vi "zoom_or_move_to_roi_grMD.vi"() -> ()   [LabVIEW 2017]
doc: "SciScan 1.2 160622"
uses:
  Custom Controls/pixel resolution enum.ctl
  GFG/GFGDisplayRefsGet.vi
  GFG/GFGfpRefGet.vi
  GFG/GFG library.lvlib
  GFG/GFGbooleanGet.vi
panel:
  out "error out 2":errorcluster
  out "error out":errorcluster
  in  "error in (no error)":errorcluster
  in  "stop":bool
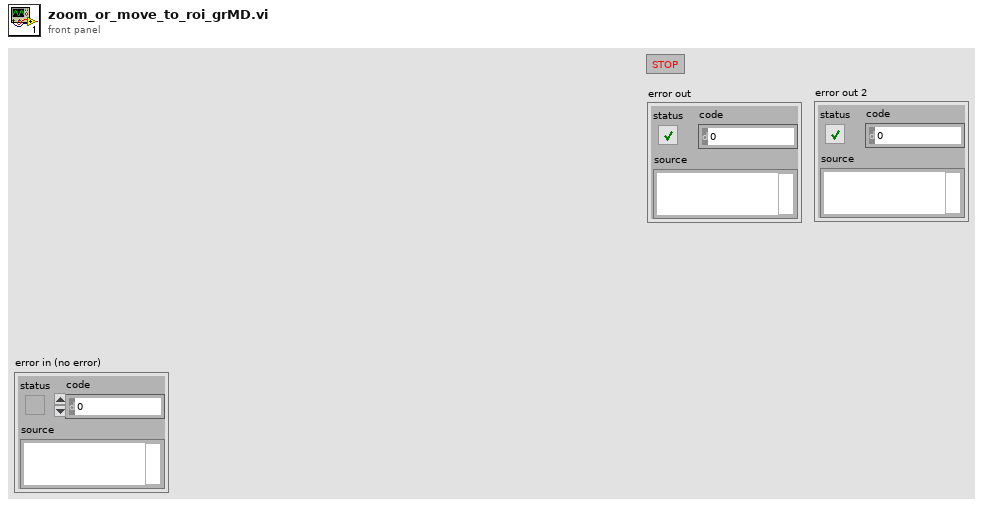
[diagram p1: front panel]
types:
  T1 = cluster{"Global Rectangle":i32[], "Contours":cluster{"Contour Type":u32, "ROI Type":u32, "Points":i32[]}[]}
  T2 = enum16{"Left Button", "Center Button", "Right Button", "Window Close"}
  T3 = cluster{"Channel 1 small":refnum<vi>, "Channel 2 small":refnum<vi>, "Channel 3 small":refnum<vi>, "Channel 4 small":refnum<vi>, "Channel 1 large":refnum<vi>, "Channel 2 large":refnum<vi>, "Channel 3 large":refnum<vi>, "Channel 4 large":refnum<vi>, "RGB overlay":refnum<vi>, "ROI Image display":refnum<vi>, "arb line scan display":refnum<vi>, "Channel 5 large":refnum<vi>}
  T4 = enum8{"Enabled", "Disabled", "Disabled and Grayed Out"}
  T5 = typedef "pixel resolution enum.ctl" = enum16{"128 x 128", "256 x 128", "256 x 256", "512 x  64", "512 x 128", "512 x 256", "512 x 512", "1024 x 512", "1024 x 1024", "arbitrary"}
  T6 = cluster{"WaveformChartRef":refnum<vi>, "DigitalRef":refnum<vi>, "ArrayRef":refnum<vi>, "TabControlRef":refnum<vi>, "EnumRef":refnum<vi>, "RingRef":refnum<vi>, "BooleanRef":refnum<vi>, "KnobRef":refnum<vi>, "SlideRef":refnum<vi>, "PathRef":refnum<vi>, "StringRef":refnum<vi>, "ComboBox":refnum<vi>, "WaveformGraphRef":refnum<vi>}
  T7 = typedef "ROI Descriptor" = cluster{"Global Rectangle":i32[], "Contours":cluster{"ID":enum32{"External", "Internal"}, "Type":u32, "Coordinates":i32[]}[]}
  T8 = cluster{"ID":enum32{"External", "Internal"}, "Type":u32, "Coordinates":i32[]}[]
  T9 = cluster{"ID":enum32{"External", "Internal"}, "Type":u32, "Coordinates":i32[]}
  T10 = cluster{"pixel resolution":variant, "x offset":variant, "x pixel size":variant, "y offset":variant, "y pixel size":variant, "y pixels":variant}
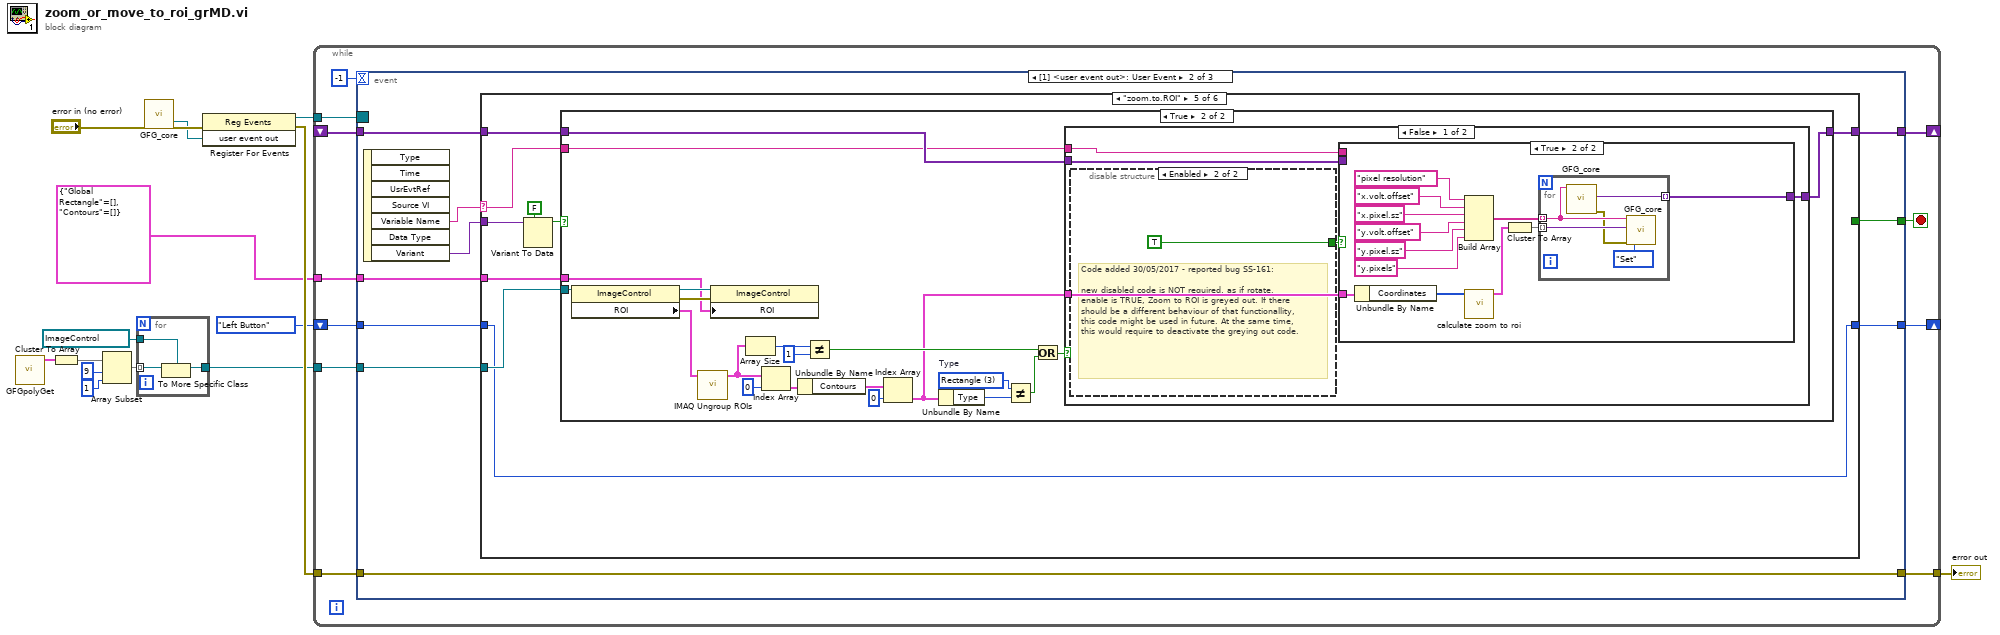
[diagram p0: block diagram]
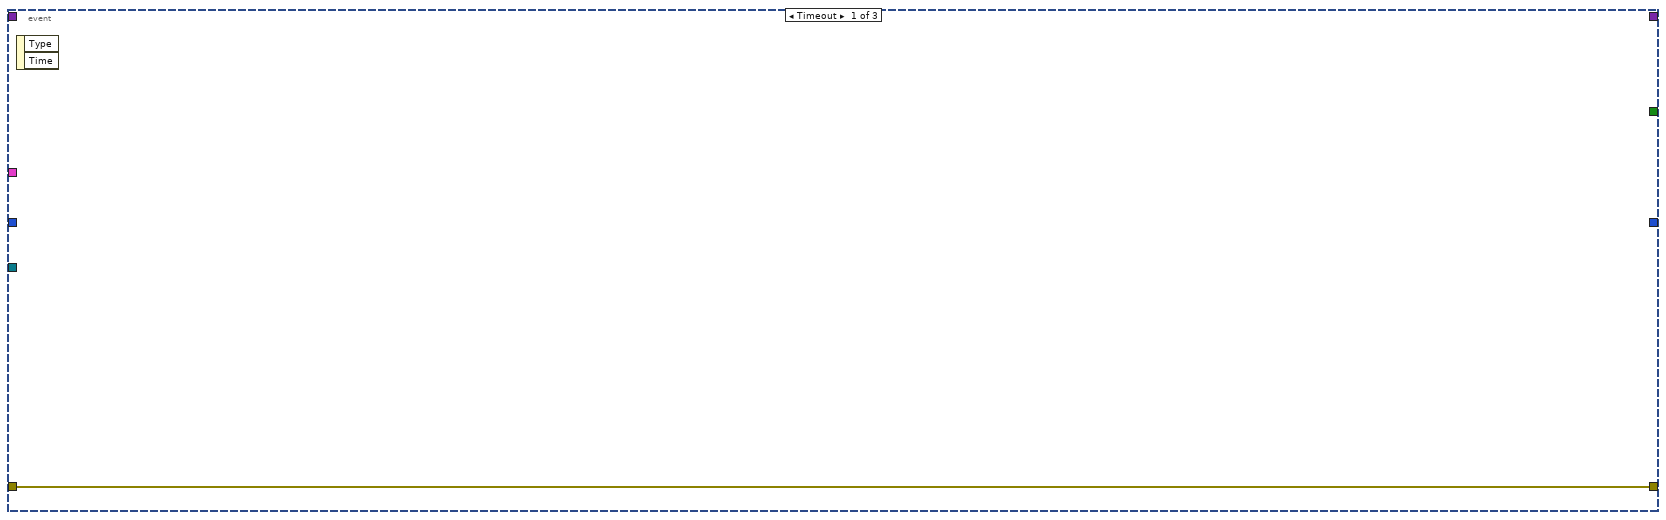
[diagram p2: hidden frame]
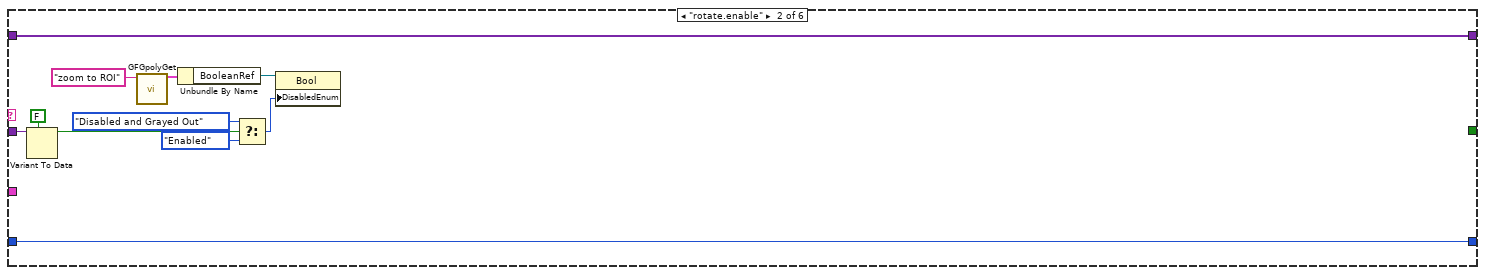
[diagram p4: hidden frame]
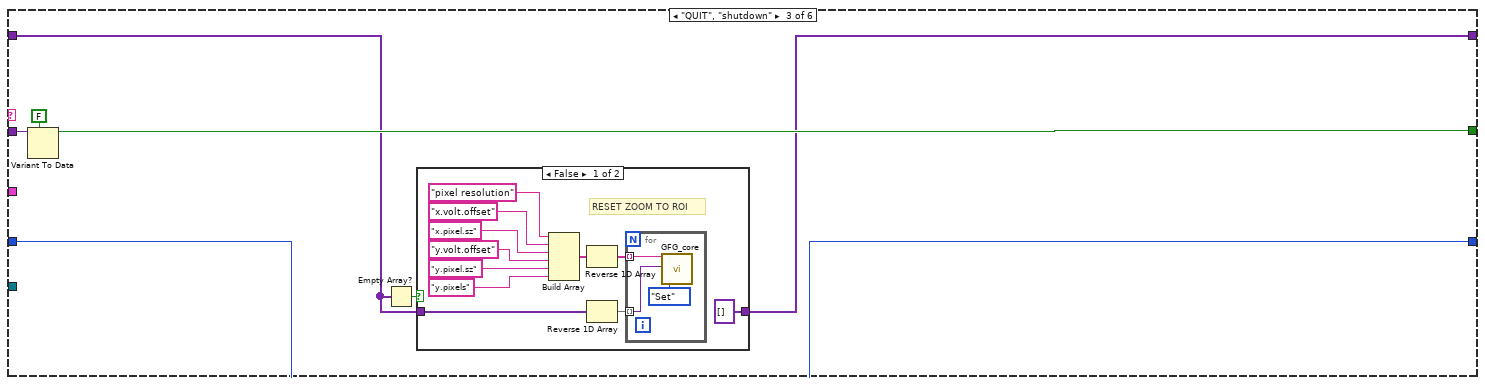
[diagram p5: hidden frame]
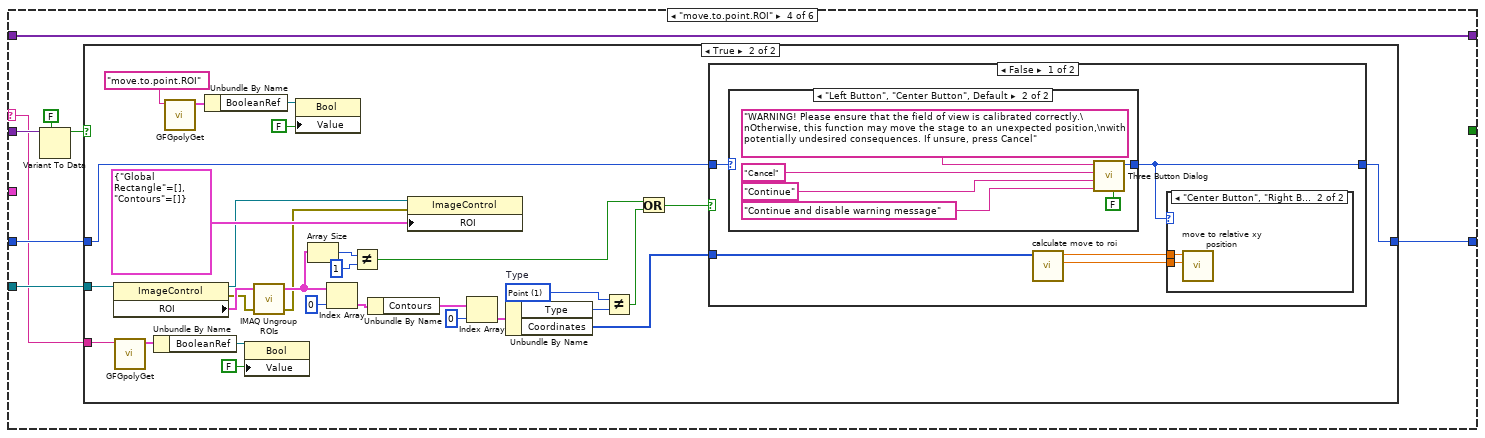
[diagram p7: hidden frame]
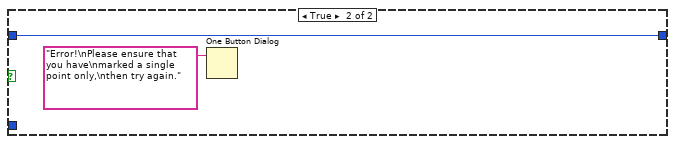
[diagram p11: hidden frame]
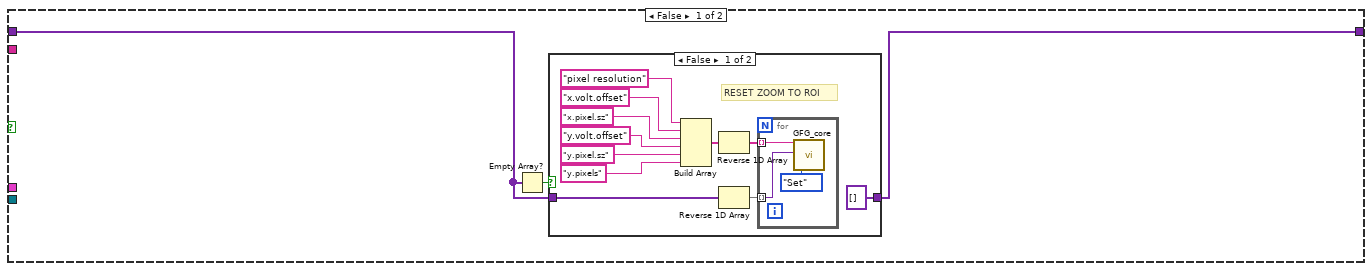
[diagram p12: hidden frame]
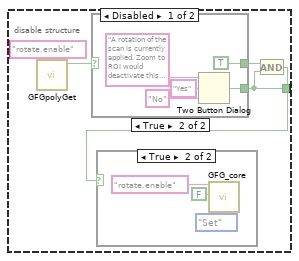
[diagram p14: hidden frame]
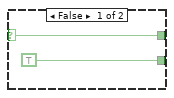
[diagram p16: hidden frame]
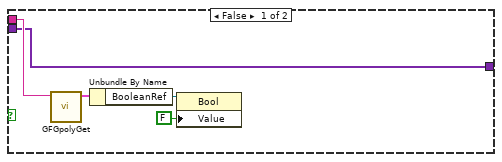
[diagram p17: hidden frame]
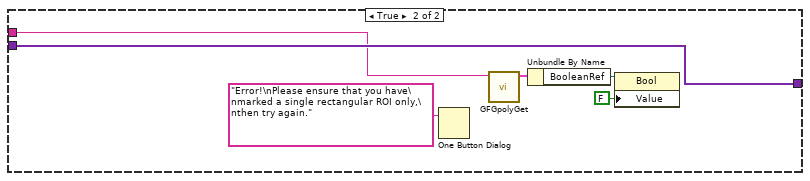
[diagram p18: hidden frame]
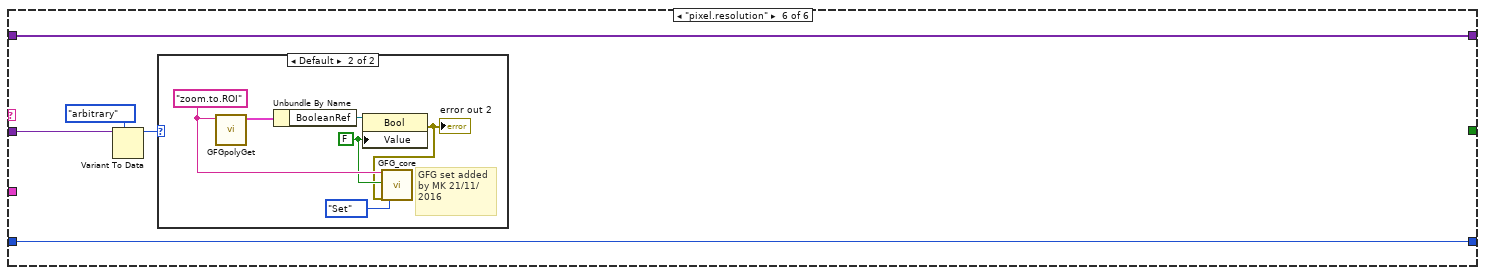
[diagram p19: hidden frame]
diagram:
  n1 = call-poly "GFGpolyGet.vi"() -> ("DisplayRefsOut(generic class)"=w10:T3)  [unwired: 10 in, 1 out]
  n2 = Cluster To Array(cluster=w10) -> (array=w13:refnum<vi>[])
  n3 = Array Subset(array=w13, index=9, length=1) -> (w12:refnum<vi>[])
  n4 = for {
    tunnel: w12 -> [w18] mode=indexing
    tunnel: refnum<vi> refnum ("arbitrary line scan display") -> [w17]
    tunnel: [w16] -> w3
    n5 = To More Specific Class(target class=w17, reference=w18) -> (specific class reference=w16:refnum<vi>)  [unwired: 1 in, 1 out]
  }
  n6 = call "GFG_core.vi"("error in (no error)"="error in (no error)") -> ("user event out"=w5:refnum<user-event>, "error out"=w6:errorcluster)  [unwired: 12 in, 5 out]
  n7 = register-events(error in=w6, w5) -> (reference out=w4:refnum<event-registration>, error out=w8:errorcluster)  [unwired: 1 in]
  n8 = while {
    tunnel: w4 -> [w29]
    tunnel: w8 -> [w27]
    tunnel: [w26] -> w9
    tunnel: w3 -> [w24]
    shift-right: [w23] -> _
    shift-left: _ -> [w22]
    shift-right: [w20] -> _
    shift-left: T2."Left Button" ("Which Button?") -> [w21]
    tunnel: T1 {"Global Rectangle"=[], "Contours"=[]} ("ROI") -> [w19]
    stop <- w28 stop-if-true
    n9 = event shown="[1] <user event out>: User Event" {
      selector: w29 -> [_ _ _]
      dyn-events: _ -> [_ _ _]
      timeout: -1 -> [_ _ _]
      tunnel: [_ w38 _] -> w28
      tunnel: w27 -> [w30 w37 _]
      tunnel: [w30 w37 _] -> w26
      tunnel: w24 -> [_ w36 _]
      tunnel: [_ w35 _] -> w23
      tunnel: w22 -> [_ w34 _]
      tunnel: w21 -> [_ w33 _]
      tunnel: [_ w32 _] -> w20
      tunnel: w19 -> [_ w31 _]
      event Timeout {
        n10 = event-data() -> ()  [unwired: 1 in, 2 out]
      }
      event User Event {
        n11 = event-data() -> ("Variable Name"=w40:string, "Variant"=w39:variant)  [unwired: 1 in, 5 out]
        n12 = case shown="\"zoom.to.ROI\"" w40 {
          selector: w40 -> [_ _ _ w76 w133 _]
          tunnel: w39 -> [_ w46 w60 w80 w136 w232]
          tunnel: [_ _ w58 _ _ _] -> w38
          tunnel: w36 -> [_ _ _ w83 w139 _]
          tunnel: [w42 w43 w57 w82 w138 w229] -> w35
          tunnel: w34 -> [w42 w43 w55 w82 w137 w229]
          tunnel: w33 -> [w41 w53 w56 w78 w132 w228]
          tunnel: [w41 w53 w56 w77 w132 w228] -> w32
          tunnel: w31 -> [_ _ _ _ w131 _]
          frame "False", Default {
          }
          frame "rotate.enable" {
            n13 = Variant To Data(type=FALSE, Variant=w46) -> (data=w44:bool)  [unwired: 1 in, 1 out]
            n14 = call-poly "GFGpolyGet.vi"("Variable Name in"="zoom to ROI") -> ("output cluster"=w51:T6)  [unwired: 9 in, 1 out]
            n15 = Unbundle By Name(w51) -> ("BooleanRef"=w50:refnum<vi>)
            n16 = Select(t=T4."Disabled and Grayed Out" ("Disabled"), s=w44, f=T4."Enabled" ("Disabled")) -> (s? t:f=w49:T4)
            n17 = property class="Bool"(reference=w50, "DisabledEnum"=w49) -> ()  [unwired: 1 in, 2 out]
          }
          frame "QUIT", "shutdown" {
            n18 = Variant To Data(type=FALSE ("want seconds? (F)"), Variant=w60) -> (data=w58:bool)  [unwired: 1 in, 1 out]
            n19 = Empty Array?(array=w55) -> (empty?=w54:bool)
            n20 = case shown="False" w54 {
              tunnel: [variant[] [] w75] -> w57
              tunnel: w55 -> [w62 w75]
              frame False {
                # "RESET ZOOM TO ROI"
                n21 = Build Array("pixel resolution" ("Variable Name in"), "x.volt.offset" ("Variable Name in"), "x.pixel.sz" ("Variable Name in"), "y.volt.offset" ("Variable Name in"), "y.pixel.sz" ("Variable Name in"), "y.pixels" ("Variable Name in")) -> (w63:string[])
                n22 = Reverse 1D Array(array=w63) -> (reversed array=w71:string[])
                n23 = Reverse 1D Array(array=w62) -> (reversed array=w70:variant[])
                n24 = for {
                  tunnel: w71 -> [w73] mode=indexing
                  tunnel: w70 -> [w72] mode=indexing
                  n25 = call "GFG_core.vi"("Variable Name in"=w73, "Variant in"=w72, "Action"=enum16{"Init", "Set", "Get", "Clear"}."Set") -> ()  [unwired: 10 in, 7 out]
                }
              }
              frame True {
                # "Do nothing, as the zoom to ROI hasn't been used yet."
              }
            }
          }
          frame "move.to.point.ROI" {
            n26 = Variant To Data(type=FALSE, Variant=w80) -> (data=w79:bool)  [unwired: 1 in, 1 out]
            n27 = case shown="True" w79 {
              tunnel: w83 -> [_ w114]
              tunnel: w78 -> [w84 w98]
              tunnel: [w84 w97] -> w77
              tunnel: w76 -> [_ w85]
              frame False {
              }
              frame True {
                w101 = u32 1 items=["No Selection", "Point", "Line", "Rectangle", "Oval", "Polygon", "Freehand Region", "Annulus", "Unused2", "Unused3", "Broken Line", "Freehand Line", "Rotated Rectangle"]  # Type
                n28 = property class="ImageControl"(reference=w114) -> (reference out=w91:refnum<vi>, error out=w90:errorcluster, "ROI"=w113:T1)  [unwired: 1 in]
                n29 = call-poly "GFGpolyGet.vi"("Variable Name in"=w85) -> ("output cluster"=w88:T6)  [unwired: 9 in, 1 out]
                n30 = Unbundle By Name(w88) -> ("BooleanRef"=w87:refnum<vi>)
                n31 = call-poly "GFGpolyGet.vi"("Variable Name in"="move.to.point.ROI") -> ("output cluster"=w95:T6)  [unwired: 9 in, 1 out]
                n32 = Unbundle By Name(w95) -> ("BooleanRef"=w94:refnum<vi>)
                n33 = property class="Bool"(reference=w87, "Value"=FALSE ("true")) -> ()  [unwired: 1 in, 2 out]
                n34 = call "IMAQ Ungroup ROIs"("error in (no error)"=w90, "ROI Descriptor"=w113) -> ("error out"=w89:errorcluster, "ROI Descriptors out"=w108:T7[])  [unwired: 2 in]
                n35 = property class="Bool"(reference=w94, "Value"=FALSE) -> ()  [unwired: 1 in, 2 out]
                n36 = Array Size(array=w108) -> (size(s)=w112:i32)
                n37 = Index Array(array=w108, index=0) -> (element=w106:T7)
                n38 = Not Equal?(x=w112, y=1) -> (x != y?=w110:bool)
                n39 = Unbundle By Name(w106) -> ("Contours"=w104:T8)
                n40 = property class="ImageControl"(reference=w91, error in=w89, "ROI"=T1 {"Global Rectangle"=[], "Contours"=[]}) -> ()  [unwired: 2 out]
                n41 = Index Array(array=w104, index=0) -> (element=w103:T9)
                n42 = Unbundle By Name(w103) -> ("Type"=w102:u32, "Coordinates"=w99:i32[])
                n43 = Not Equal?(x=w101, y=w102) -> (x != y?=w100:bool)
                n44 = Or(x=w110, y=w100) -> (x .or. y?=w109:bool)
                n45 = case shown="False" w109 {
                  tunnel: w99 -> [w119 _]
                  tunnel: w98 -> [w118 w129]
                  tunnel: [w115 w129] -> w97
                  frame False {
                    n46 = case shown="\"Left Button\", \"Center Button\", Default" w118 {
                      selector: w118 -> [w120 _]
                      tunnel: [w120 w123] -> w115
                      frame "Right Button" {
                      }
                      frame "Left Button", "Center Button", Default {
                        n47 = call <vilib>:"Three Button Dialog.vi"("Allow user to close window? (TRUE)"=FALSE, "Right Button Text (\"Cancel\")"="Continue and disable warning message" ("Center Button Text (\"No\")"), "Center Button Text (\"No\")"="Continue" ("Left Button Text (\"Yes\")"), "Left Button Text (\"Yes\")"="Cancel" ("Right Button Text (\"Cancel\")"), "message"="WARNING! Please ensure that the field of view is calibrated correctly.\nOtherwise, this function may move the stage to an unexpected position,\nwith potentially undesired consequences. If unsure, press Cancel") -> ("Which Button?"=w123:T2)  [unwired: 6 in]
                      }
                    }
                    n48 = call "calculate move to roi.vi"("Coordinates"=w119) -> ("setY"=w116:dbl, "setX"=w117:dbl)  [unwired: 9 in]
                    n49 = case shown="\"Center Button\", \"Right Button\"" w115 {
                      tunnel: w117 -> [_ w128]
                      tunnel: w116 -> [_ w127]
                      frame "Left Button", Default {
                      }
                      frame "Center Button", "Right Button" {
                        n50 = call "move to relative xy position.vi"("setY"=w127, "setX"=w128) -> ()  [unwired: 10 in]
                      }
                    }
                  }
                  frame True {
                    n51 = One Button Dialog(message="Error!\nPlease ensure that you have\nmarked a single point only,\nthen try again.") -> ()  [unwired: 1 in, 1 out]
                  }
                }
              }
            }
          }
          frame "zoom.to.ROI" {
            n52 = Variant To Data(type=FALSE, Variant=w136) -> (data=w134:bool)  [unwired: 1 in, 1 out]
            n53 = case shown="True" w134 {
              tunnel: w139 -> [_ w178]
              tunnel: [w140 w163] -> w138
              tunnel: w137 -> [w141 w162]
              tunnel: w133 -> [_ w159]
              tunnel: w131 -> [_ w158]
              frame False {
                n54 = Empty Array?(array=w141) -> (empty?=w142:bool)
                n55 = case shown="False" w142 {
                  tunnel: [variant[] [] w157] -> w140
                  tunnel: w141 -> [w144 w157]
                  frame False {
                    # "RESET ZOOM TO ROI"
                    n56 = Build Array("pixel resolution" ("Variable Name in"), "x.volt.offset" ("Variable Name in"), "x.pixel.sz" ("Variable Name in"), "y.volt.offset" ("Variable Name in"), "y.pixel.sz" ("Variable Name in"), "y.pixels" ("Variable Name in")) -> (w145:string[])
                    n57 = Reverse 1D Array(array=w145) -> (reversed array=w153:string[])
                    n58 = Reverse 1D Array(array=w144) -> (reversed array=w152:variant[])
                    n59 = for {
                      tunnel: w153 -> [w155] mode=indexing
                      tunnel: w152 -> [w154] mode=indexing
                      n60 = call "GFG_core.vi"("Variable Name in"=w155, "Variant in"=w154, "Action"=enum16{"Init", "Set", "Get", "Clear"}."Set") -> ()  [unwired: 10 in, 7 out]
                    }
                  }
                  frame True {
                    # "Do nothing, as the zoom to ROI hasn't been used yet."
                  }
                }
              }
              frame True {
                w166 = u32 3 items=["No Selection", "Point", "Line", "Rectangle", "Oval", "Polygon", "Freehand Region", "Annulus", "Unused2", "Unused3", "Broken Line", "Freehand Line", "Rotated Rectangle"]  # Type
                n61 = property class="ImageControl"(reference=w178) -> (reference out=w161:refnum<vi>, error out=w160:errorcluster, "ROI"=w177:T1)  [unwired: 1 in]
                n62 = call "IMAQ Ungroup ROIs"("ROI Descriptor"=w177) -> ("ROI Descriptors out"=w172:T7[])  [unwired: 3 in, 1 out]
                n63 = property class="ImageControl"(reference=w161, error in=w160, "ROI"=w158) -> ()  [unwired: 2 out]
                n64 = Array Size(array=w172) -> (size(s)=w176:i32)
                n65 = Index Array(array=w172, index=0) -> (element=w170:T7)
                n66 = Unbundle By Name(w170) -> ("Contours"=w168:T8)
                n67 = Not Equal?(x=w176, y=1) -> (x != y?=w174:bool)
                n68 = Index Array(array=w168, index=0) -> (element=w164:T9)
                n69 = Unbundle By Name(w164) -> ("Type"=w167:u32)
                n70 = Not Equal?(x=w166, y=w167) -> (x != y?=w165:bool)
                n71 = Or(x=w174, y=w165) -> (x .or. y?=w173:bool)
                n72 = case shown="False" w173 {
                  tunnel: w164 -> [w183 _]
                  tunnel: [w182 w227] -> w163
                  tunnel: w162 -> [w179 w227]
                  tunnel: w159 -> [w180 w226]
                  frame False {
                    n73 = disable-structure shown="Enabled" {
                      disable-tunnel: [w185 TRUE ("T button?")] -> w181
                      frame Disabled {
                        n74 = call-poly "GFGpolyGet.vi"("Variable Name in"="rotate.enable" ("message")) -> ("Boolean Value OUT"=w187:bool)  [unwired: 9 in, 1 out]
                        n75 = case shown="True" w187 {
                          selector: w187 -> [w192 _]
                          tunnel: [TRUE ("T button?") w195] -> w185
                          tunnel: [w192 TRUE] -> w186
                          frame False {
                          }
                          frame True {
                            n76 = Two Button Dialog(message="A rotation of the scan is currently applied. Zoom to ROI would deactivate this rotation. Do you want to proceed?", 1:"No" ("F button name (\"Cancel\")"), 2:"Yes" ("T button name (\"OK\")")) -> (T button?=w195:bool)
                          }
                        }
                        n77 = And(x=w186, y=w185) -> (x .and. y?=w184:bool)
                        n78 = case shown="True" w184 {
                          frame False {
                          }
                          frame True {
                            n79 = call "GFG_core.vi"("Variable Name in"="rotate.enable" ("message"), "Variant in"=FALSE ("T button?"), "Action"=enum16{"Init", "Set", "Get", "Clear"}."Set") -> ()  [unwired: 10 in, 7 out]
                          }
                        }
                      }
                      frame Enabled {
                        # "Code added 30/05/2017 - reported bug SS-161:\n\nnew disabled code is NOT required, as if rotate.enable is TRUE, Zoom to ROI is greyed out. If there should be a different behaviour of that functionallity, this code might be used in future. At the same time, this would require to deactivate the greying out code."
                      }
                    }
                    n80 = case shown="True" w181 {
                      tunnel: w183 -> [_ w216]
                      tunnel: [w200 w215] -> w182
                      tunnel: w180 -> [w201 _]
                      tunnel: w179 -> [w200 _]
                      frame False {
                        n81 = call-poly "GFGpolyGet.vi"("Variable Name in"=w201) -> ("output cluster"=w204:T6)  [unwired: 9 in, 1 out]
                        n82 = Unbundle By Name(w204) -> ("BooleanRef"=w203:refnum<vi>)
                        n83 = property class="Bool"(reference=w203, "Value"=FALSE ("true")) -> ()  [unwired: 1 in, 2 out]
                      }
                      frame True {
                        n84 = Unbundle By Name(w216) -> ("Coordinates"=w214:i32[])
                        n85 = Build Array("pixel resolution" ("Variable Name in"), "x.volt.offset" ("Variable Name in"), "x.pixel.sz" ("Variable Name in"), "y.volt.offset" ("Variable Name in"), "y.pixel.sz" ("Variable Name in"), "y.pixels" ("Variable Name in")) -> (w207:string[])
                        n86 = call "calculate zoom to roi.vi"("Coordinates"=w214) -> ("output cluster"=w208:T10)  [unwired: 10 in]
                        n87 = Cluster To Array(cluster=w208) -> (array=w206:variant[])
                        n88 = for {
                          tunnel: w207 -> [w219] mode=indexing
                          tunnel: w206 -> [w220] mode=indexing
                          tunnel: [w218] -> w215 mode=indexing
                          n89 = call "GFG_core.vi"("Variable Name in"=w219) -> ("Variant Out"=w218:variant, "error out"=w217:errorcluster)  [unwired: 12 in, 5 out]
                          n90 = call "GFG_core.vi"("Variable Name in"=w219, "Variant in"=w220, "error in (no error)"=w217, "Action"=enum16{"Init", "Set", "Get", "Clear"}."Set") -> ()  [unwired: 9 in, 7 out]
                        }
                      }
                    }
                  }
                  frame True {
                    n91 = One Button Dialog(message="Error!\nPlease ensure that you have\nmarked a single rectangular ROI only,\nthen try again.") -> ()  [unwired: 1 in, 1 out]
                    n92 = call-poly "GFGpolyGet.vi"("Variable Name in"=w226) -> ("output cluster"=w225:T6)  [unwired: 9 in, 1 out]
                    n93 = Unbundle By Name(w225) -> ("BooleanRef"=w224:refnum<vi>)
                    n94 = property class="Bool"(reference=w224, "Value"=FALSE ("true")) -> ()  [unwired: 1 in, 2 out]
                  }
                }
              }
            }
          }
          frame "pixel.resolution" {
            n95 = Variant To Data(type=pixel_resolution_enum."arbitrary" ("pixel resolution"), Variant=w232) -> (data=w230:T5)  [unwired: 1 in, 1 out]
            n96 = case shown="Default" w230 {
              frame "arbitrary" {
              }
              frame Default {
                w234 = FALSE
                w235 = "zoom.to.ROI"
                # "GFG set added by MK 21/11/2016"
                n97 = call-poly "GFGpolyGet.vi"("Variable Name in"=w235) -> ("output cluster"=w238:T6)  [unwired: 9 in, 1 out]
                n98 = Unbundle By Name(w238) -> ("BooleanRef"=w237:refnum<vi>)
                n99 = property class="Bool"(reference=w237, "Value"=w234) -> (error out=w233:errorcluster)  [unwired: 1 in, 1 out]
                "error out 2" <- w233
                n100 = call "GFG_core.vi"("Variable Name in"=w235, "Variant in"=w234, "error in (no error)"=w233, "Action"=enum16{"Init", "Set", "Get", "Clear"}."Set") -> ()  [unwired: 9 in, 7 out]
              }
            }
          }
        }
      }
      event "stop": Value Change {
        n101 = event-data() -> ()  [unwired: 1 in, 5 out]
        n102 = call "getVIname.vi"() -> ("VI name"=w239:string)  [unwired: 19 in]
        n103 = call "SendShutdownCommand.vi"("Source VI"=w239) -> ()  [unwired: 11 in]
      }
    }
  }
  "error out" <- w9
